vi "ClassRenamer_Interface.vi"(9 "EventsIn":T1, 10 "Events":T2) -> ()   [LabVIEW 2014, in "ClassRenamer.lvclass"]
uses:
  ClassRenamer.lvclass
  GCMCore/Providers/Veritech_GCM/Support/Framework/_Plugins/_LVCMPlugin/GCMPlugin_EventsOut.ctl
  GCMCore/Providers/Veritech_GCM/Support/Framework/_Plugins/_LVCMPlugin/GCMPlugin_EventsIn.ctl
  GCMCore/Providers/Veritech_GCM/Support/Framework/_Plugins/GCMPlugin/GCMPlugin.lvclass
panel:
  in  "Rename":bool
  in  "Change Members Names":bool=TRUE
  in  "Change Controls Names":bool=TRUE
  in  "Output String":string
  in  "Input String":string
  in  "New Path":path
  in  "Replace String":string
  in  "Search String":string
  in  "New Name":string
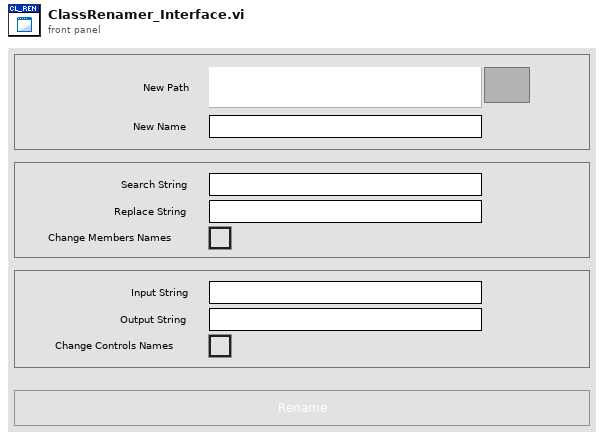
[diagram p1: front panel]
types:
  T1 = typedef "GCMPlugin.lvclass/GCMPlugin_EventsIn.ctl" = cluster{"Stop":refnum<user-event>, "ItemSelected":refnum<user-event>, "ItemDeselected":refnum<user-event>, "PluginActivated":refnum<user-event>, "PluginDeactivated":refnum<user-event>}
  T2 = typedef "GCMPlugin.lvclass/GCMPlugin_EventsOut.ctl" = cluster{"ItemEdited":refnum<user-event>}
  T3 = enum8{"Enabled", "Disabled", "Disabled and Grayed Out"}
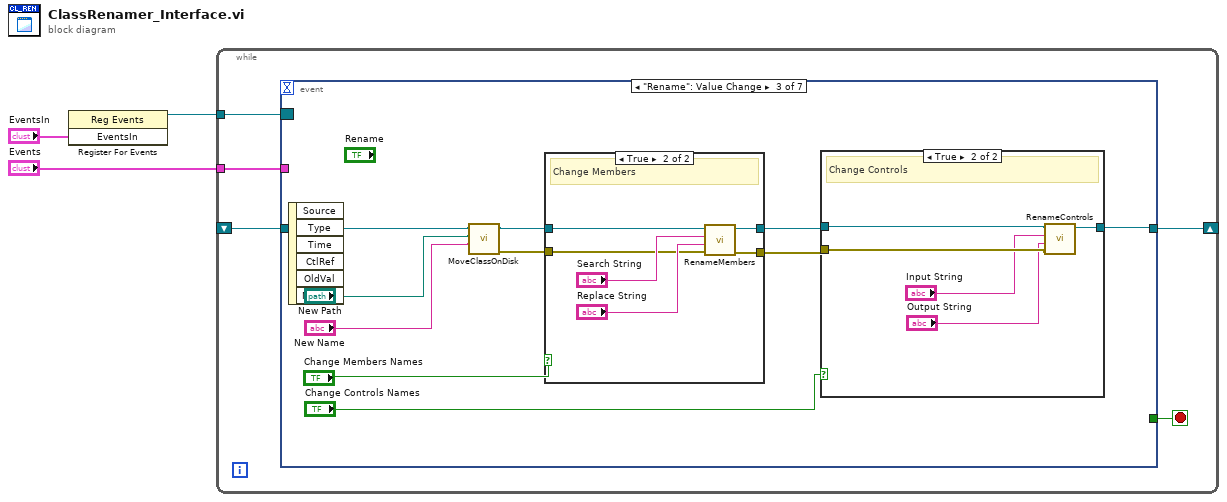
[diagram p0: block diagram]
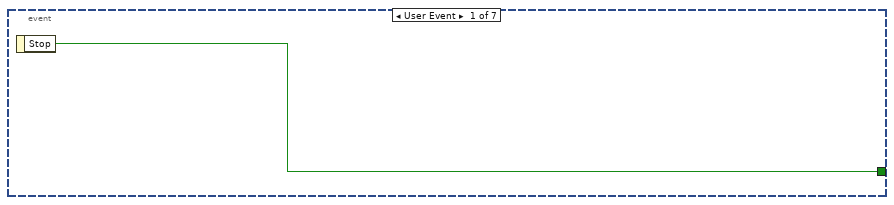
[diagram p2: hidden frame]
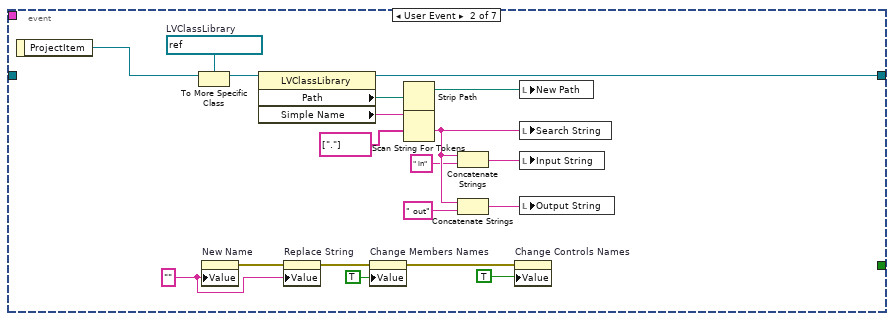
[diagram p3: hidden frame]
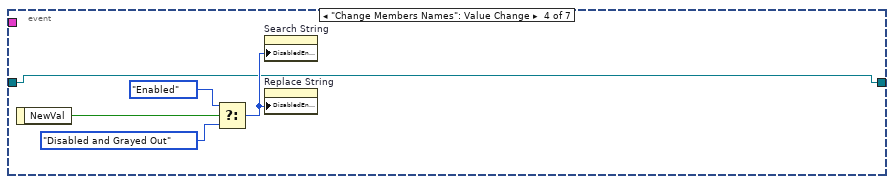
[diagram p6: hidden frame]
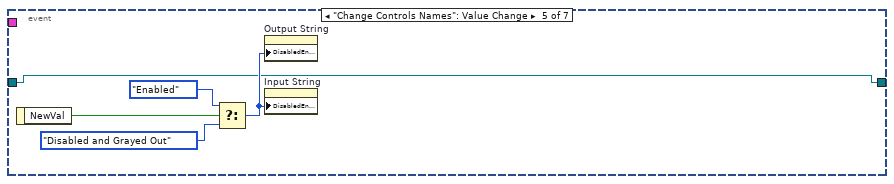
[diagram p7: hidden frame]
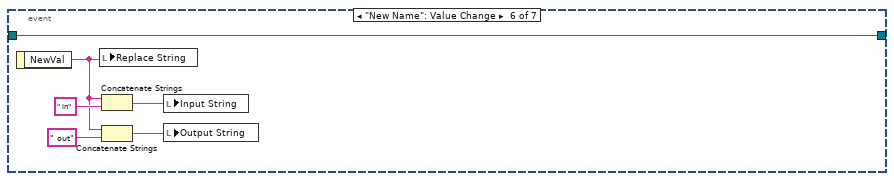
[diagram p8: hidden frame]
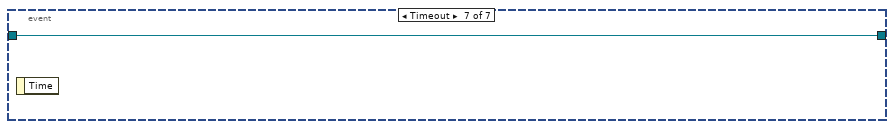
[diagram p9: hidden frame]
diagram:
  n1 = register-events("EventsIn") -> (reference out=w2:refnum<event-registration>)  [unwired: 2 in, 1 out]
  n2 = while {
    tunnel: w2 -> [w8]
    tunnel: "Events" -> [w7]
    shift-right: [w4] -> _
    shift-left: _ -> [w5]
    stop <- w6 stop-if-true
    n3 = event shown="[2] \"Rename\": Value Change" {
      selector: w8 -> [_ _ _ _ _ _ _]
      dyn-events: _ -> [_ _ _ _ _ _ _]
      timeout: _ -> [_ _ _ _ _ _ _]
      tunnel: w7 -> [_ _ _ _ _ _ _]
      tunnel: [w9 _ _ _ _ _ _] -> w6
      tunnel: w5 -> [_ _ w38 w53 w58 w63 w69]
      tunnel: [_ w10 w29 w53 w58 w63 w69] -> w4
      event User Event {
        n4 = event-data() -> ("Stop"=w9:bool)  [unwired: 1 in]
      }
      event User Event {
        w12 = refnum<vi> refnum  # LVClassLibrary
        w27 = ""
        n5 = event-data() -> ("ProjectItem"=w11:refnum<vi>)  [unwired: 1 in]
        n6 = To More Specific Class(target class=w12, reference=w11) -> (specific class reference=w13:refnum<vi>)  [unwired: 1 in, 1 out]
        n7 = property on="New Name" class="Str"("Value"=w27) -> (error out=w26:errorcluster)  [unwired: 2 in, 1 out]
        n8 = property class="LVClassLibrary"(reference=w13) -> (reference out=w10:refnum<vi>, "Path"=w16:path, "Simple Name"=w14:string)  [unwired: 1 in, 1 out]
        n9 = property on="Replace String" class="Str"(error in=w26, "Value"=w27) -> (error out=w28:errorcluster)  [unwired: 1 in, 1 out]
        n10 = property on="Change Members Names" class="Bool (strict)"(error in=w28, "Value"=TRUE ("Value (Signaling)")) -> (error out=w24:errorcluster)  [unwired: 1 in, 1 out]
        n11 = Strip Path(path=w16) -> (stripped path=w17:path)  [unwired: 1 out]
        n12 = Scan String For Tokens(7:string[] ["."] ("operators (none)"), 9:w14) -> (1:w20:string)  [unwired: 4 in, 3 out]
        n13 = Concatenate Strings(w20, " in" ("string")) -> (w21:string)
        n14 = Concatenate Strings(w20, " out" ("string")) -> (w22:string)
        n15 = property on="Change Controls Names" class="Bool (strict)"(error in=w24, "Value"=TRUE ("Change Members Names")) -> ()  [unwired: 1 in, 2 out]
        n16 = local write "New Path"(w17) -> ()
        n17 = local write "Search String"(w20) -> ()
        n18 = local write "Input String"(w21) -> ()
        n19 = local write "Output String"(w22) -> ()
      }
      event "Rename": Value Change {
        n20 = event-data() -> ()  [unwired: 1 in, 6 out]
        n21 = call "MoveClassOnDisk.vi"("NewName"="New Name", "NewPath"="New Path", "LVClassLibrary Refnum"=w38) -> ("error out"=w34:errorcluster, "Library Refnum out"=w37:refnum<vi>)  [unwired: 7 in]
        n22 = case shown="True" "Change Members Names" {
          tunnel: w37 -> [w46 w52]
          tunnel: w34 -> [w45 w49]
          tunnel: [w46 w48] -> w33
          tunnel: [w45 w47] -> w32
          frame False {
            # "Nothing"
          }
          frame True {
            # "Change Members"
            n23 = call "RenameMembers.vi"("error in (no error)"=w49, "ReplaceString"="Replace String", "SearchString"="Search String", "LVClassLibrary Refnum"=w52) -> ("error out"=w47:errorcluster, "Library Refnum out"=w48:refnum<vi>)  [unwired: 6 in]
          }
        }
        n24 = case shown="True" "Change Controls Names" {
          tunnel: w33 -> [w39 w44]
          tunnel: w32 -> [_ w43]
          tunnel: [w39 w40] -> w29
          frame False {
            # "Nothing"
          }
          frame True {
            # "Change Controls"
            n25 = call "RenameControls.vi"("error in (no error)"=w43, "Output String"="Output String", "Input String"="Input String", "LVClassLibrary Refnum"=w44) -> ("Library Refnum out"=w40:refnum<vi>)  [unwired: 6 in, 1 out]
          }
        }
      }
      event "Change Members Names": Value Change {
        n26 = event-data() -> ("NewVal"=w57:bool)  [unwired: 1 in]
        n27 = Select(t=T3."Enabled" ("Disabled"), s=w57, f=T3."Disabled and Grayed Out" ("Disabled")) -> (s? t:f=w54:T3)
        n28 = property on="Search String" class="Str"("DisabledEnum"=w54) -> ()  [unwired: 2 in, 2 out]
        n29 = property on="Replace String" class="Str"("DisabledEnum"=w54) -> ()  [unwired: 2 in, 2 out]
      }
      event "Change Controls Names": Value Change {
        n30 = event-data() -> ("NewVal"=w62:bool)  [unwired: 1 in]
        n31 = Select(t=T3."Enabled" ("Disabled"), s=w62, f=T3."Disabled and Grayed Out" ("Disabled")) -> (s? t:f=w59:T3)
        n32 = property on="Output String" class="Str"("DisabledEnum"=w59) -> ()  [unwired: 2 in, 2 out]
        n33 = property on="Input String" class="Str"("DisabledEnum"=w59) -> ()  [unwired: 2 in, 2 out]
      }
      event "New Name": Value Change {
        n34 = event-data() -> ("NewVal"=w64:string)  [unwired: 1 in]
        n35 = local write "Replace String"(w64) -> ()
        n36 = Concatenate Strings(w64, " in" ("string")) -> (w67:string)
        n37 = Concatenate Strings(w64, " out" ("string")) -> (w68:string)
        n38 = local write "Input String"(w67) -> ()
        n39 = local write "Output String"(w68) -> ()
      }
      event Timeout {
        n40 = event-data() -> ()  [unwired: 1 in, 1 out]
      }
    }
  }
